vi "Hyper Terminal.vi"() -> ()   [LabVIEW 2018]
uses:
  <vilib>/event_ctls.llb/eventvkey.ctl
  <vilib>/Instr/_visa.llb/Select Event Type.ctl
  <vilib>/Instr/_visa.llb/VISA Configure Serial Port (Instr).vi
panel:
  out "Time Stamp":timestamp format="%<%H:%M:%S\n%d/%m/%Y>T"
  in  "Exit":bool
  in  "Clear Screen":bool
  in  "Data":string
  in  "Display Style":T1(ring)
  in  "Flow Control":T2(ring)
  in  "Stop Bits":u16(ring)=10 items=["1.0"=10, "1.5"=15, "2.0"=20]
  in  "Parity":enum16{"None", "Odd", "Even", "Mark", "Space"}(ring)
  in  "Data Bits":u16=8 min=5 max=8 step=1
  in  "Baud Rate":i32(ring)=9600 items=["110"=110, "300"=300, "600"=600, "1200"=1200, "2400"=2400, "4800"=4800, "9600"=9600, "14400"=14400, "19200"=19200, "38400"=38400, "56000"=56000, "115200"=115200, "128000"=128000, "256000"=256000]
  in  "Com Port":string(combo)
  in  "Autoscroll":bool
  in  "CR=> CR/LF":bool
  in  "Local Echo":bool
  in  "Autowrap":bool
  in  "File Send":bool
  in  "File Log":bool
  out "Boolean":bool
  in  "Connect":bool
  out "Quit":bool
  in  "error in (no error)":errorcluster
  out "error out":errorcluster
  # "Hyper Terminal"
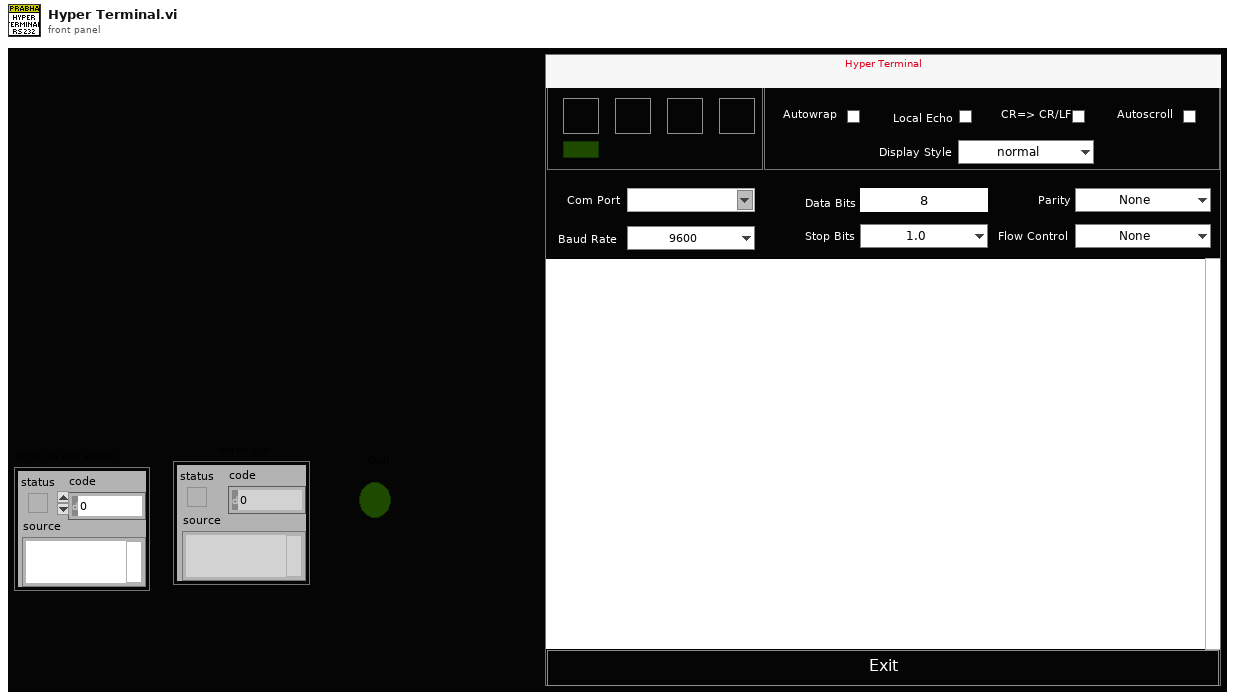
[diagram p1: front panel]
types:
  T1 = enum32{"normal", "backslash '\\' codes", "password", "hex"}
  T2 = enum16{"None", "XON/XOFF", "RTS/CTS", "XON/XOFF & RTS/CTS", "DTR/DSR", "XON/XOFF & DTR/DSR"}
  T3 = cluster{"Data":string, "VISA":refnum<visa-resource-name>, "refnum":refnum<file>, "Log File":bool}
  T4 = typedef "eventvkey.ctl" = enum16{"ASCII", "Enter", "Return", "Shift", "Ctrl", "Alt", "Cmd", "Opt", "Caps", "NumLock", "Clear", "Break", "Up", "Down", "Left", "Right", "Insert", "Delete", "Home", "End", "PageUp", "PageDown", "Escape", "Help", "Pause", "ScrollLock", "F1", "F2", "F3", "F4", "F5", "F6", "F7", "F8", "F9", "F10", "F11", "F12", "F13", "F14", "F15", "F16", "F17", "F18", "F19", "F20", "F21", "F22", "F23", "F24", "Play", "VolumeUp", "VolumeDown", "Mute", "Two Byte Char"}
  T5 = enum16{"open", "replace", "create", "open or create", "replace or create", "replace or create with confirmation"}
  T6 = typedef "Select Event Type.ctl" = u32
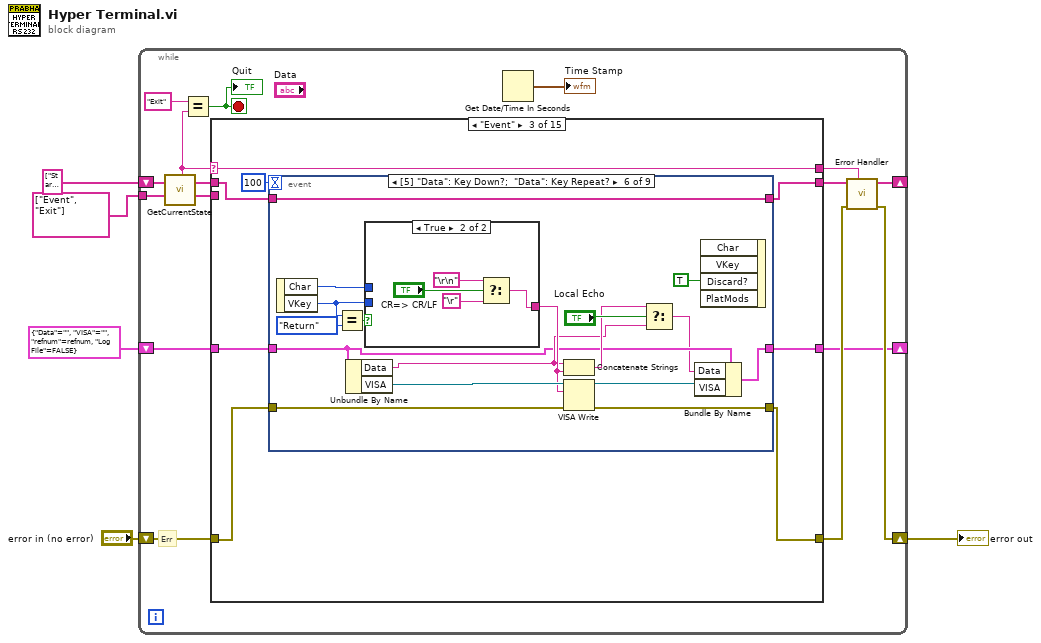
[diagram p0: block diagram]
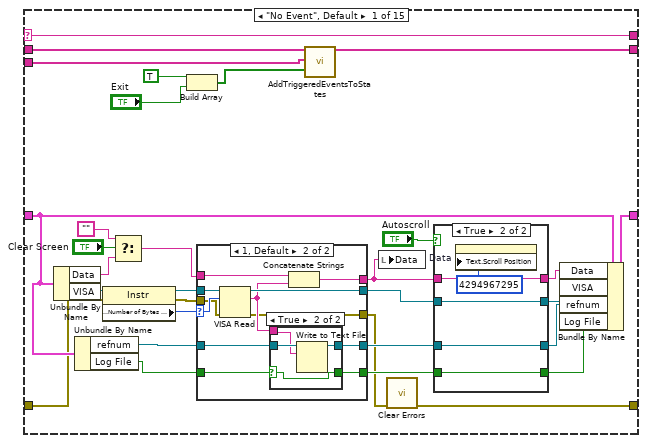
[diagram p2: hidden frame]
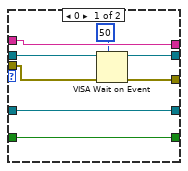
[diagram p4: hidden frame]
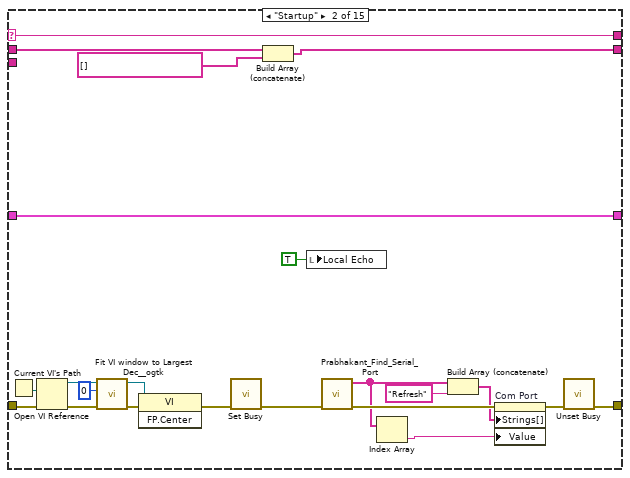
[diagram p6: hidden frame]
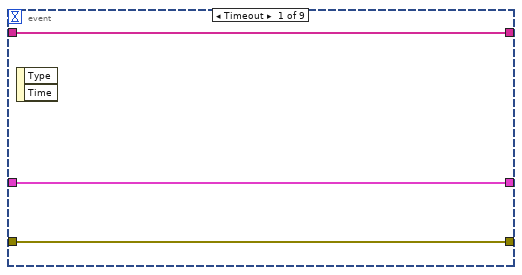
[diagram p7: hidden frame]
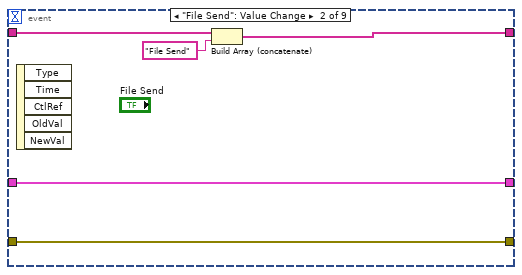
[diagram p8: hidden frame]
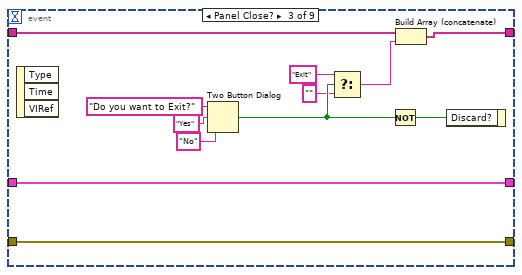
[diagram p9: hidden frame]
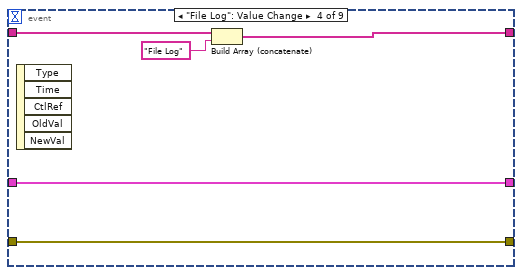
[diagram p10: hidden frame]
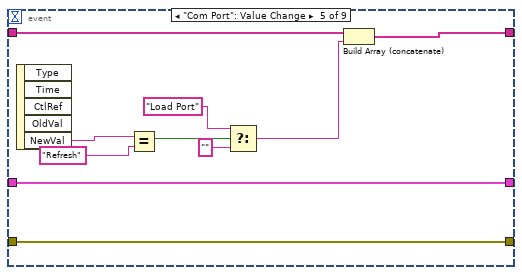
[diagram p11: hidden frame]
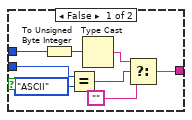
[diagram p12: hidden frame]
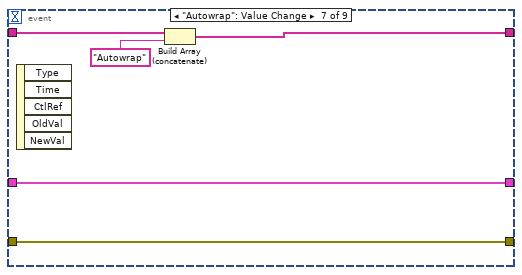
[diagram p13: hidden frame]
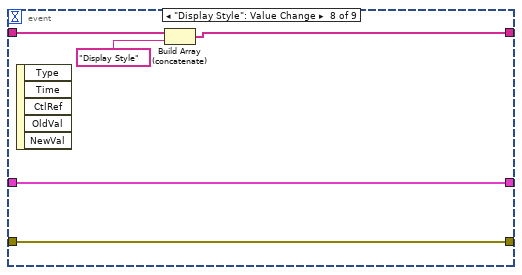
[diagram p14: hidden frame]
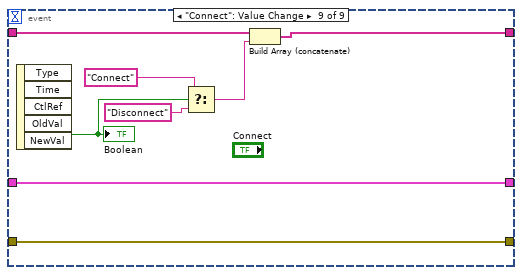
[diagram p15: hidden frame]
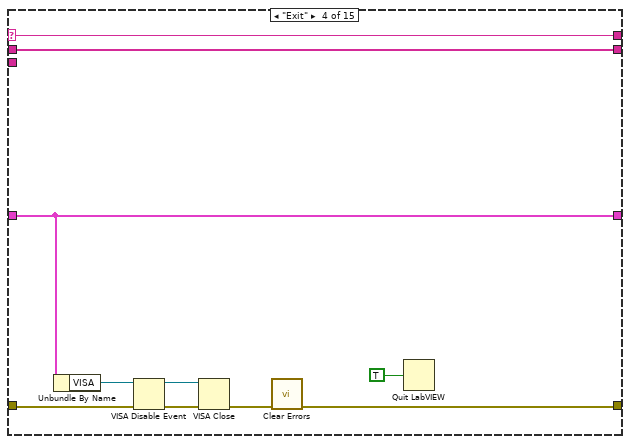
[diagram p16: hidden frame]
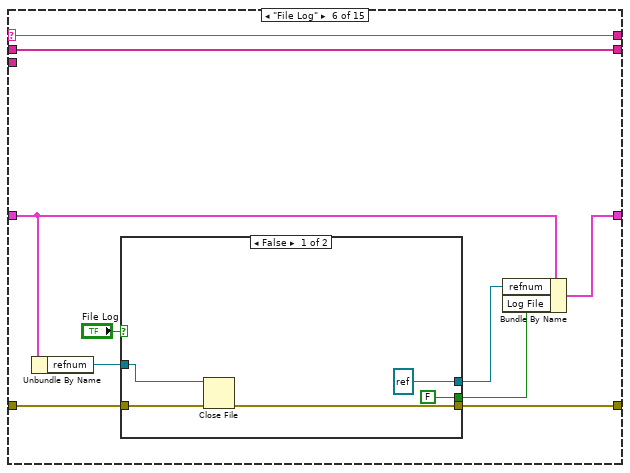
[diagram p18: hidden frame]
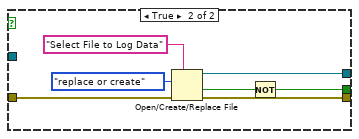
[diagram p19: hidden frame]
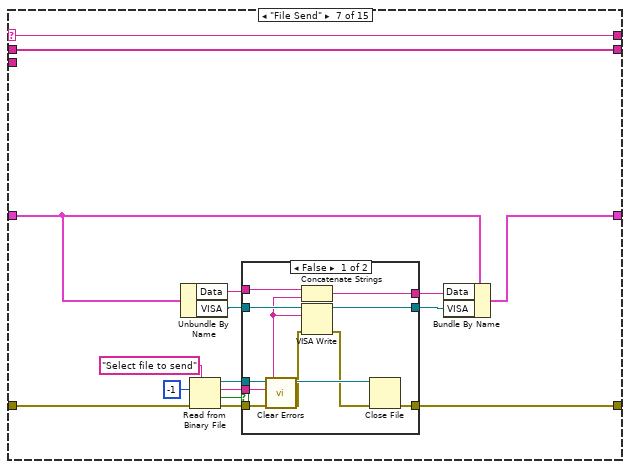
[diagram p20: hidden frame]
diagram:
  n1 = while {
    shift-right: [w13] -> _
    shift-left: string[] ["Startup"] ("State Array Out") -> [w20]
    tunnel: string[] ["Event", "Exit"] ("State Array Out") -> [w18]
    shift-right: [w10] -> w4
    shift-left: "error in (no error)" -> [w14]
    shift-right: [w7] -> _
    shift-left: T3 {"Data"="", "VISA"="", "refnum"=refnum, "Log File"=FALSE} -> [w8]
    stop <- w15 stop-if-true
    # "Err"
    n2 = call "GetCurrentState.vi"("State Array In"=w20) -> ("Current State"=w16:string, "State Array Out"=w19:string[])  [unwired: 1 in, 16 out]
    n3 = Equal?(x="Exit", y=w16) -> (x = y?=w15:bool)
    "Quit" <- w15
    n4 = case shown="\"Event\"" w16 {
      selector: w16 -> [w49 w105 w116 w208 w210 w221 w249 w269 w276 w283 w294 w318 w329 w334 w348]
      tunnel: w19 -> [w51 w107 w115 w207 w212 w222 w250 w270 w277 w285 w295 w319 w330 w333 w347]
      tunnel: [w46 w106 w114 w207 w212 w222 w250 w270 w277 w285 w295 w319 w330 w333 w347] -> w12
      tunnel: w18 -> [w50 _ _ _ _ _ _ _ _ _ _ _ _ _ _]
      tunnel: [w22 w87 w109 w200 w211 w219 w237 w266 w272 w284 w286 w298 w321 w332 errorcluster {"status"=FALSE, "code"=0, "source"=""} ("error in (no error)")] -> w9
      tunnel: w14 -> [w24 w99 w110 w206 w211 w220 w248 w267 w274 w284 w287 w317 w328 w332 w346]
      tunnel: [w49 w105 w116 w208 w210 w221 w249 w269 w276 w283 w294 w318 w329 w334 w348] -> w11
      tunnel: w8 -> [w27 w93 w112 w202 w209 w214 w242 w268 w275 w282 w293 w300 w323 w331 w335]
      tunnel: [w26 w93 w111 w202 w209 w217 w241 w268 w275 w282 w293 w299 w322 w331 w335] -> w7
      frame "No Event", Default {
        n5 = Unbundle By Name(w27) -> ("Data"=w38:string, "VISA"=w45:refnum<visa-resource-name>)
        n6 = Unbundle By Name(w27) -> ("refnum"=w42:refnum<file>, "Log File"=w41:bool)
        n7 = property class="Instr"(reference=w45, error in=w24) -> (reference out=w43:refnum<visa-resource-name>, error out=w25:errorcluster, "Serial Settings:Number of Bytes at Serial Port"=w44:u32)
        n8 = Select(t="", s="Clear Screen", f=w38) -> (s? t:f=w37:string)
        n9 = Build Array(TRUE, "Exit") -> (w48:bool[])
        n10 = case shown="1, Default" w44 {
          selector: w44 -> [_ w79]
          tunnel: w43 -> [w65 w80]
          tunnel: w37 -> [w68 w77]
          tunnel: [w64 w78] -> w36
          tunnel: w42 -> [w67 w76]
          tunnel: w41 -> [w66 w73]
          tunnel: [w67 w74] -> w31
          tunnel: [w66 w72] -> w30
          tunnel: [w68 w71] -> w35
          tunnel: w25 -> [w62 w70]
          tunnel: [w61 w69] -> w23
          frame 0 {
            n11 = VISA Wait on Event(7:u32 50 ("timeout (0)"), 8:w62, 11:w65) -> (0:w61:errorcluster, 3:w64:refnum<visa-resource-name>)  [unwired: 2 in, 2 out]
          }
          frame 1, Default {
            n12 = VISA Read(VISA resource name=w80, byte count=w79, error in (no error)=w70) -> (VISA resource name out=w78:refnum<visa-resource-name>, read buffer=w75:string, error out=w69:errorcluster)  [unwired: 1 out]
            n13 = case shown="True" w73 {
              selector: w73 -> [w81 w83]
              tunnel: w76 -> [w82 w86]
              tunnel: w75 -> [_ w85]
              tunnel: [w82 w84] -> w74
              tunnel: [w81 w83] -> w72
              frame False {
              }
              frame True {
                n14 = Write to Text File(file (use dialog)=w86, text=w85) -> (refnum out=w84:refnum<file>)  [unwired: 2 in, 2 out]
              }
            }
            n15 = Concatenate Strings(w77, w75) -> (w71:string)
          }
        }
        n16 = call "AddTriggeredEventsToStates.vi"("State Array In"=w51, "Event List"=w50, "Event Triggers Array"=w48) -> ("State Array Out"=w46:string[])  [unwired: 16 out]
        n17 = local write "Data"(w35) -> ()
        n18 = call <vilib>:"Clear Errors.vi"("error in (no error)"=w23) -> ("error out"=w22:errorcluster)  [unwired: 5 in, 1 out]
        n19 = case shown="True" "Autoscroll" {
          tunnel: w36 -> [w54 w59]
          tunnel: w35 -> [w55 w58]
          tunnel: [w54 w59] -> w32
          tunnel: [w55 w58] -> w33
          tunnel: w31 -> [w53 w57]
          tunnel: [w53 w57] -> w29
          tunnel: w30 -> [w52 w56]
          tunnel: [w52 w56] -> w28
          frame False {
          }
          frame True {
            n20 = property on="Data" class="Str"("Text.Scroll Position"=u32 4294967295) -> ()  [unwired: 2 in, 2 out]
          }
        }
        n21 = Bundle By Name(cluster=w27, "Data"=w33, "VISA"=w32, "refnum"=w29, "Log File"=w28) -> (w26:T3)
      }
      frame "Startup" {
        n22 = Current VI's Path() -> (path=w102:path)
        n23 = Open VI Reference(vi path=w102, error in (no error)=w99) -> (vi reference=w103:refnum<vi>, error out=w98:errorcluster)  [unwired: 4 out]
        n24 = call "Fit VI window to Largest Dec__ogtk.vi"("error in (no error)"=w98, "border spacing (2 px)"=0, "VI Ref (calling VI)"=w103) -> ("error out"=w101:errorcluster, "dup VI Ref"=w100:refnum<vi>)  [unwired: 3 out]
        n25 = invoke class="VI" method="FP.Center"(reference=w100, error in=w101) -> (error out=w97:errorcluster)  [unwired: 1 in, 2 out]
        n26 = call <vilib>:"Set Busy.vi"("error in (no error)"=w97) -> ("error out"=w88:errorcluster)  [unwired: 9 in, 1 out]
        n27 = Build Array (concatenate)(w107, string[] [] ("State Array Out")) -> (w106:string[])
        n28 = local write "Local Echo"(TRUE ("Local Echo")) -> ()
        n29 = call "Prabhakant_Find_Serial_Port.vi"("error in (no error)"=w88) -> ("error out"=w95:errorcluster, "Array"=w91:string[])  [unwired: 9 in]
        n30 = Index Array(array=w91) -> (element=w96:string)  [unwired: 1 in]
        n31 = Build Array (concatenate)(w91, "Refresh") -> (w90:string[])
        n32 = property on="Com Port" class="CmbBox"(error in=w95, "Strings[]"=w90, "Value"=w96) -> (error out=w94:errorcluster)  [unwired: 1 in, 1 out]
        n33 = call <vilib>:"Unset Busy.vi"("error in (no error)"=w94) -> ("error out"=w87:errorcluster)  [unwired: 10 in]
      }
      frame "Event" {
        n34 = event shown="[5] \"Data\": Key Down?;  \"Data\": Key Repeat?" {
          selector: _ -> [_ _ _ _ _ _ _ _ _]
          dyn-events: _ -> [_ _ _ _ _ _ _ _ _]
          timeout: 100 -> [_ _ _ _ _ _ _ _ _]
          tunnel: w115 -> [w119 w124 w136 w141 w151 w168 w185 w190 w198]
          tunnel: [w119 w121 w133 w138 w145 w168 w184 w189 w197] -> w114
          tunnel: w112 -> [w118 w123 w135 w140 w150 w158 w182 w187 w192]
          tunnel: [w118 w123 w135 w140 w150 w157 w182 w187 w192] -> w111
          tunnel: w110 -> [w117 w122 w134 w139 w149 w153 w181 w186 w191]
          tunnel: [w117 w122 w134 w139 w149 w152 w181 w186 w191] -> w109
          event Timeout {
            n35 = event-data() -> ()  [unwired: 1 in, 2 out]
          }
          event "File Send": Value Change {
            n36 = event-data() -> ()  [unwired: 1 in, 5 out]
            n37 = Build Array (concatenate)(w124, "File Send") -> (w121:string[])
          }
          event Panel Close? {
            n38 = event-data() -> ()  [unwired: 1 in, 3 out]
            n39 = Two Button Dialog(message="Do you want to Exit?", 1:"No" ("F button name (\"Cancel\")"), 2:"Yes" ("T button name (\"OK\")")) -> (T button?=w128:bool)
            n40 = Select(t="Exit" ("x"), s=w128, f="") -> (s? t:f=w125:string)
            n41 = Not(x=w128) -> (.not. x?=w129:bool)
            n42 = Build Array (concatenate)(w136, w125) -> (w133:string[])
            n43 = event-data("Discard?"=w129) -> ()  [unwired: 1 in, 1 out]
          }
          event "File Log": Value Change {
            n44 = event-data() -> ()  [unwired: 1 in, 5 out]
            n45 = Build Array (concatenate)(w141, "File Log") -> (w138:string[])
          }
          event "Com Port": Value Change {
            n46 = event-data() -> ("NewVal"=w148:string)  [unwired: 1 in, 4 out]
            n47 = Equal?(x=w148, y="Refresh") -> (x = y?=w146:bool)
            n48 = Select(t="Load Port", s=w146, f="") -> (s? t:f=w142:string)
            n49 = Build Array (concatenate)(w151, w142) -> (w145:string[])
          }
          event "Data": Key Down?; "Data": event type 3.0.x8000000b {
            n50 = event-data() -> ("Char"=w167:i16, "VKey"=w164:T4)  [unwired: 1 in]
            n51 = Equal?(x=w164, y=eventvkey."Return") -> (x = y?=w166:bool)
            n52 = Unbundle By Name(w158) -> ("Data"=w159:string, "VISA"=w163:refnum<visa-resource-name>)
            n53 = case shown="True" w166 {
              tunnel: w167 -> [w176 _]
              tunnel: w164 -> [w174 _]
              tunnel: [w169 w177] -> w162
              frame False {
                n54 = To Unsigned Byte Integer(number=w176) -> (unsigned 8bit integer=w175:u8)
                n55 = Equal?(x=w174, y=eventvkey."ASCII") -> (x = y?=w171:bool)
                n56 = Type Cast(x=w175) -> (*(type *) &x=w172:string)  [unwired: 1 in]
                n57 = Select(t=w172, s=w171, f="") -> (s? t:f=w169:string)
              }
              frame True {
                n58 = Select(t="\r\n", s="CR=> CR/LF", f="\r") -> (s? t:f=w177:string)
              }
            }
            n59 = Concatenate Strings(w159, w162) -> (w160:string)
            n60 = VISA Write(VISA resource name=w163, write buffer=w162, error in (no error)=w153) -> (VISA resource name out=w155:refnum<visa-resource-name>, error out=w152:errorcluster)  [unwired: 1 out]
            n61 = Select(t=w160, s="Local Echo", f=w159) -> (s? t:f=w156:string)
            n62 = Bundle By Name(cluster=w158, "Data"=w156, "VISA"=w155) -> (w157:T3)
            n63 = event-data("Discard?"=TRUE) -> ()  [unwired: 4 in, 1 out]
          }
          event "Autowrap": Value Change {
            n64 = event-data() -> ()  [unwired: 1 in, 5 out]
            n65 = Build Array (concatenate)(w185, "Autowrap" ("x")) -> (w184:string[])
          }
          event "Display Style": Value Change {
            n66 = event-data() -> ()  [unwired: 1 in, 5 out]
            n67 = Build Array (concatenate)(w190, "Display Style" ("x")) -> (w189:string[])
          }
          event "Connect": Value Change {
            n68 = event-data() -> ("NewVal"=w196:bool)  [unwired: 1 in, 4 out]
            "Boolean" <- w196
            n69 = Select(t="Connect", s=w196, f="Disconnect") -> (s? t:f=w194:string)
            n70 = Build Array (concatenate)(w198, w194) -> (w197:string[])
          }
        }
      }
      frame "Exit" {
        n71 = Unbundle By Name(w202) -> ("VISA"=w201:refnum<visa-resource-name>)
        n72 = VISA Disable Event(8:w206, 11:w201) -> (0:w205:errorcluster, 3:w203:refnum<visa-resource-name>)  [unwired: 2 in]
        n73 = VISA Close(VISA resource name=w203, error in (no error)=w205) -> (error out=w204:errorcluster)
        n74 = call <vilib>:"Clear Errors.vi"("error in (no error)"=w204) -> ("error out"=w200:errorcluster)  [unwired: 5 in, 1 out]
        n75 = Quit LabVIEW(quit? (T)=TRUE) -> ()
      }
      frame "---------------Below are UI Events---------------" {
      }
      frame "File Log" {
        n76 = Unbundle By Name(w214) -> ("refnum"=w213:refnum<file>)
        n77 = case shown="False" "File Log" {
          tunnel: w220 -> [w227 w233]
          tunnel: [w226 w232] -> w219
          tunnel: [refnum<file> refnum ("refnum out") w231] -> w216
          tunnel: [FALSE w229] -> w215
          tunnel: w213 -> [w225 _]
          frame False {
            n78 = Close File(refnum=w225, error in=w227) -> (error out=w226:errorcluster)  [unwired: 1 out]
          }
          frame True {
            n79 = Open/Create/Replace File(error in=w233, prompt="Select File to Log Data", operation (0:open)=T5."replace or create") -> (refnum out=w231:refnum<file>, cancelled=w230:bool, error out=w232:errorcluster)  [unwired: 3 in]
            n80 = Not(x=w230) -> (.not. x?=w229:bool)
          }
        }
        n81 = Bundle By Name(cluster=w214, "refnum"=w216, "Log File"=w215) -> (w217:T3)
      }
      frame "File Send" {
        n82 = Unbundle By Name(w242) -> ("Data"=w245:string, "VISA"=w244:refnum<visa-resource-name>)
        n83 = Read from Binary File(7:"Select file to send" ("prompt (Open existing file)"), 8:w248, 10:-1 ("count (1)")) -> (0:w238:errorcluster, 1:w235:bool, 2:w243:string, 3:w236:refnum<file>)  [unwired: 3 in]
        n84 = case shown="False" w235 {
          tunnel: w245 -> [w260 w264]
          tunnel: w244 -> [w259 w263]
          tunnel: w243 -> [w258 _]
          tunnel: [w257 w264] -> w240
          tunnel: [w256 w263] -> w239
          tunnel: w238 -> [w253 w262]
          tunnel: [w255 w261] -> w237
          tunnel: w236 -> [w254 _]
          frame False {
            n85 = call <vilib>:"Clear Errors.vi"("error in (no error)"=w253) -> ("error out"=w251:errorcluster)  [unwired: 5 in, 1 out]
            n86 = Concatenate Strings(w260, w258) -> (w257:string)
            n87 = VISA Write(VISA resource name=w259, write buffer=w258, error in (no error)=w251) -> (VISA resource name out=w256:refnum<visa-resource-name>, error out=w252:errorcluster)  [unwired: 1 out]
            n88 = Close File(refnum=w254, error in=w252) -> (error out=w255:errorcluster)  [unwired: 1 out]
          }
          frame True {
            n89 = call <vilib>:"Clear Errors.vi"("error in (no error)"=w262) -> ("error out"=w261:errorcluster)  [unwired: 5 in, 1 out]
          }
        }
        n90 = Bundle By Name(cluster=w242, "Data"=w240, "VISA"=w239) -> (w241:T3)
      }
      frame "Display Style" {
        n91 = property on="Data" class="Str"(error in=w267, "Display Style"="Display Style") -> (error out=w266:errorcluster)  [unwired: 1 in, 1 out]
      }
      frame "Autowrap" {
        n92 = property on="Data" class="Str"(error in=w274, "WrappingEnabled"="Autowrap") -> (error out=w273:errorcluster)  [unwired: 1 in, 1 out]
        n93 = case shown="False" "Autowrap" {
          tunnel: w273 -> [w280 w281]
          tunnel: [w279 w281] -> w272
          frame False {
            n94 = property on="Data" class="Str"(error in=w280, "HScrollVis"=TRUE ("Horizontal Scrollbar Visible")) -> (error out=w279:errorcluster)  [unwired: 1 in, 1 out]
          }
          frame True {
          }
        }
      }
      frame "---------------Below are Subroutine states---------------" {
      }
      frame "Load Port" {
        n95 = call "Prabhakant_Find_Serial_Port.vi"("error in (no error)"=w287) -> ("error out"=w291:errorcluster, "Array"=w289:string[])  [unwired: 9 in]
        n96 = Index Array(array=w289) -> (element=w292:string)  [unwired: 1 in]
        n97 = Build Array (concatenate)(w289, "Refresh") -> (w288:string[])
        n98 = property on="Com Port" class="CmbBox"(error in=w291, "Strings[]"=w288, "Value"=w292) -> (error out=w286:errorcluster)  [unwired: 1 in, 1 out]
      }
      frame "Connect" {
        w302 = T6 1073684533 items=["Service Request"=1073684491, "Trigger"=3221168138, "Clear"=1073684493, "VXI Signal"=1073684512, "VXI/VME Interrupt"=3221168161, "VXI/VME Sysfail"=1073684509, "VXI/VME Sysreset"=1073684510, "GPIB CIC"=1073684498, "GPIB Talk"=1073684499, "GPIB Listen"=1073684500, "PXI Interrupt"=1073684514, "Serial Break"=1073684515, "Serial TermChar"=1073684516, "Serial CTS"=1073684521, "Serial DSR"=1073684522, "Serial DCD"=1073684524, "Serial RI"=1073684526, "Serial Character"=1073684533, "USB Interrupt"=1073684535, "All Enabled"=1073709055] ("Event Type")
        n99 = Unbundle By Name(w300) -> ("VISA"=w316:refnum<visa-resource-name>)
        n100 = VISA Disable Event(8:w317, 11:w316) -> (0:w315:errorcluster, 3:w313:refnum<visa-resource-name>)  [unwired: 2 in]
        n101 = VISA Close(VISA resource name=w313, error in (no error)=w315) -> (error out=w314:errorcluster)
        n102 = call <vilib>:"Clear Errors.vi"("error in (no error)"=w314) -> ("error out"=w312:errorcluster)  [unwired: 5 in, 1 out]
        n103 = call-poly "VISA Configure Serial Port"("VISA resource name"="Com Port", "Enable Termination\nChar (T)"=FALSE ("Enable Termination\nChar (T)"), "baud rate (9600)"="Baud Rate", "data bits (8)"="Data Bits", "parity (0:none)"="Parity", "error in (no error)"=w312, "stop bits (10: 1 bit)"="Stop Bits", "flow control (0:none)"="Flow Control") -> ("VISA resource name out"=w304:refnum<visa-resource-name>, "error out"=w303:errorcluster)  [unwired: 6 in]
        n104 = VISA Enable Event(8:w303, 10:w302, 11:w304) -> (0:w298:errorcluster, 3:w301:refnum<visa-resource-name>)  [unwired: 1 in]
        n105 = Unbundle By Name(w298) -> ("status"=w297:bool)
        n106 = Bundle By Name(cluster=w300, "VISA"=w301) -> (w299:T3)
        n107 = Not(x=w297) -> (.not. x?=w296:bool)
        n108 = local write "Connect"(w296) -> ()
        n109 = local write "Boolean"(w296) -> ()
      }
      frame "Disconnect" {
        n110 = Unbundle By Name(w323) -> ("VISA"=w327:refnum<visa-resource-name>)
        n111 = VISA Disable Event(8:w328, 11:w327) -> (0:w326:errorcluster, 3:w324:refnum<visa-resource-name>)  [unwired: 2 in]
        n112 = VISA Close(VISA resource name=w324, error in (no error)=w326) -> (error out=w325:errorcluster)
        n113 = call <vilib>:"Clear Errors.vi"("error in (no error)"=w325) -> ("error out"=w321:errorcluster)  [unwired: 5 in, 1 out]
        n114 = Bundle By Name(cluster=w323, "VISA"=refnum<visa-resource-name> refnum) -> (w322:T3)
      }
      frame "---------------Below are Error Handling VIs---------------" {
      }
      frame "Error" {
        # "Add More Error Handling If Required Like\nWriting Error Log Files\nExiting Application\nSending Auto mails\netc etc."
        n115 = Call Chain() -> (call chain=w340:string[])
        n116 = for {
          tunnel: w340 -> [w351] mode=indexing
          shift-right: [w349] -> w337
          shift-left: "" -> [w352]
          n117 = Concatenate Strings(w352, w351, " -> ") -> (w349:string)
        }
        n118 = Unbundle By Name(w346) -> ("code"=w341:i32, "source"=w344:string)
        n119 = Match Pattern(string=w344, regular expression=":") -> (before substring=w338:string, after substring=w342:string)  [unwired: 3 out]
        n120 = Format Into String(format string="Error Occured In\"%s\" state of \"%s\" VI\nError Code: %d\nError Description: \"%s\"", w338, w337, w341, w342) -> ()  [unwired: 2 in, 2 out]
      }
    }
    n121 = Get Date/Time In Seconds() -> (seconds since 1Jan1904=→"Time Stamp":timestamp)
    n122 = call "Error Handler.vi"("Current State"=w11, "error in (no error)"=w9, "Msg Queue In"=w12) -> ("error out"=w10:errorcluster, "Msg Queue Out"=w13:string[])  [unwired: 7 out]
  }
  "error out" <- w4
